vi "GetSampleRate.vi"(8 "error in (no error)":errorcluster, 11 "VISA Refnum in":refnum<visa-resource-name>) -> (0 "error out":errorcluster, 2 "SampleRate(S/sec)":dbl, 3 "VISA Refnum out":refnum<visa-resource-name>)   [LabVIEW 2013]
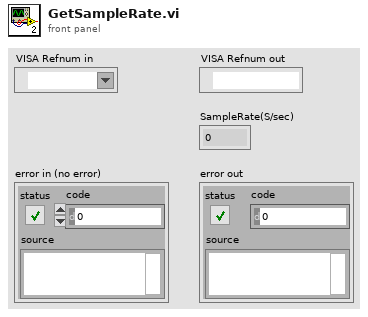
[diagram p1: front panel]
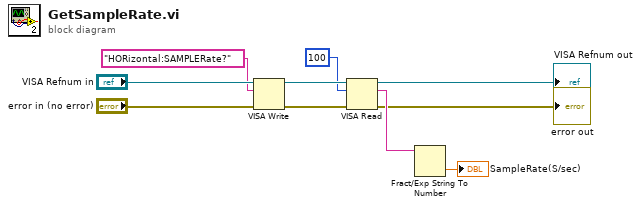
[diagram p0: block diagram]
diagram:
  n1 = VISA Write(VISA resource name="VISA Refnum in", write buffer="HORizontal:SAMPLERate?", error in (no error)="error in (no error)") -> (VISA resource name out=w4:refnum<visa-resource-name>, error out=w2:errorcluster)  [unwired: 1 out]
  n2 = VISA Read(VISA resource name=w4, byte count=u32 100, error in (no error)=w2) -> (VISA resource name out=→"VISA Refnum out":refnum<visa-resource-name>, read buffer=w7:string, error out=→"error out":errorcluster)  [unwired: 1 out]
  n3 = Fract/Exp String To Number(string=w7) -> (number=→"SampleRate(S/sec)":dbl)  [unwired: 3 in, 1 out]
